vi "VMI_save_Files_backup.vi"(0 "appended path":path=path "C:/Users/Parkes/Documents/GitHub/Camera-Acquire_Labview/120416aa", 1 "ChangeFile":bool, 3 "Hist_full":dbl[][][](array[numeric]), 4 "Image Info":T1={"X size"=782.0, "Y size"=582.0, "Centroiding"=1.0}, 5 "Histogram_array":i32[][](array[numeric]), 6 "Current File Date":string, 7 "Remote Save?":bool, 9 "Collection Information":T3[](array[typedef]), 10 "Save":bool[](array[boolean]), 11 "error in (no error)":errorcluster, 12 "Remote_path":path=path "C:/Users/Parkes/Documents/GitHub/Camera-Acquire_Labview/120416aa", 13 "Peaks":T2[](array[typedef])) -> (8 "Remote_path\n 2":path[](array[path]), 15 "error out":errorcluster)   [LabVIEW 2020]
uses:
  Type defs/FileAcq_v1_Ctrl.ctl
  Type defs/VMI_peak_out.ctl
  Type defs/Image_info.ctl
  <vilib>/Utility/file.llb/Write Delimited Spreadsheet (string).vi
panel:
  out "size(s) 3":i32
  out "size(s) 2":i32[](array[numeric])
  out "size(s)":i32[](array[numeric])
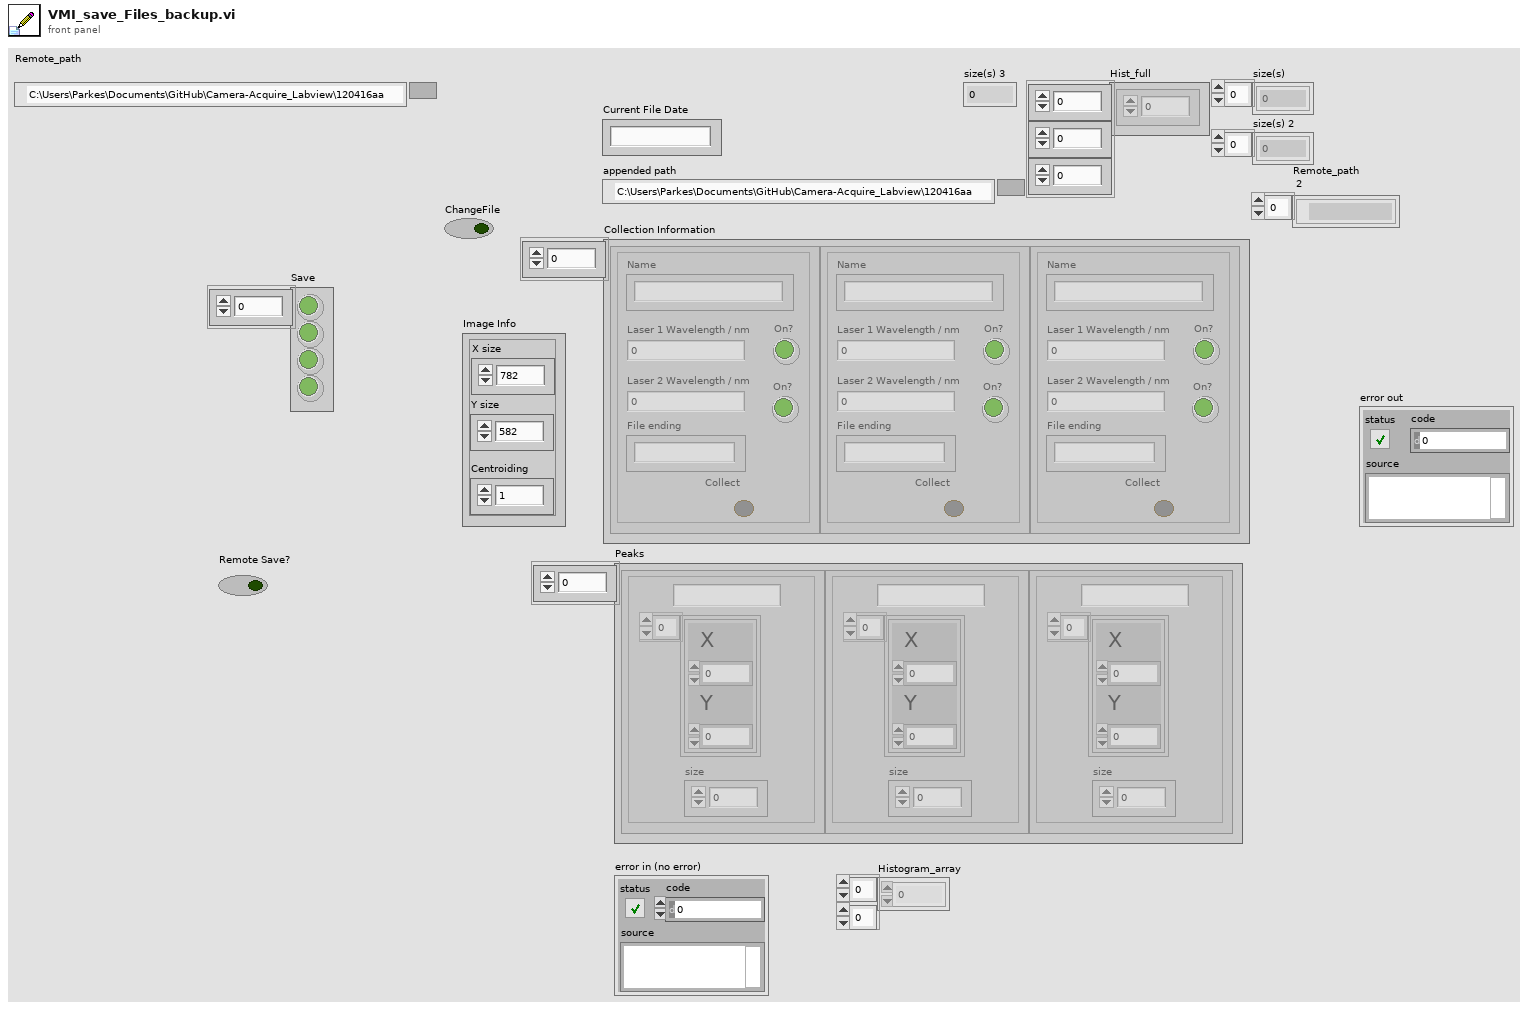
[diagram p1: front panel]
types:
  T1 = typedef "Image_info.ctl" = cluster{"X size":dbl, "Y size":dbl, "Centroiding":dbl}
  T2 = typedef "VMI_peak_out.ctl" = cluster{"Peaks":cluster{"X":sgl, "Y":sgl}[], "size":i32, "Title":string}
  T3 = typedef "FileAcq_v1_Ctrl.ctl" = cluster{"Type":string, "LaserWave1":dbl, "Shutter1":bool, "LaserWave2":dbl, "Shutter2":bool, "FileEnd":string, "Collect":bool}
  T4 = enum16{"open", "replace", "create", "open or create", "replace or create", "replace or create with confirmation"}
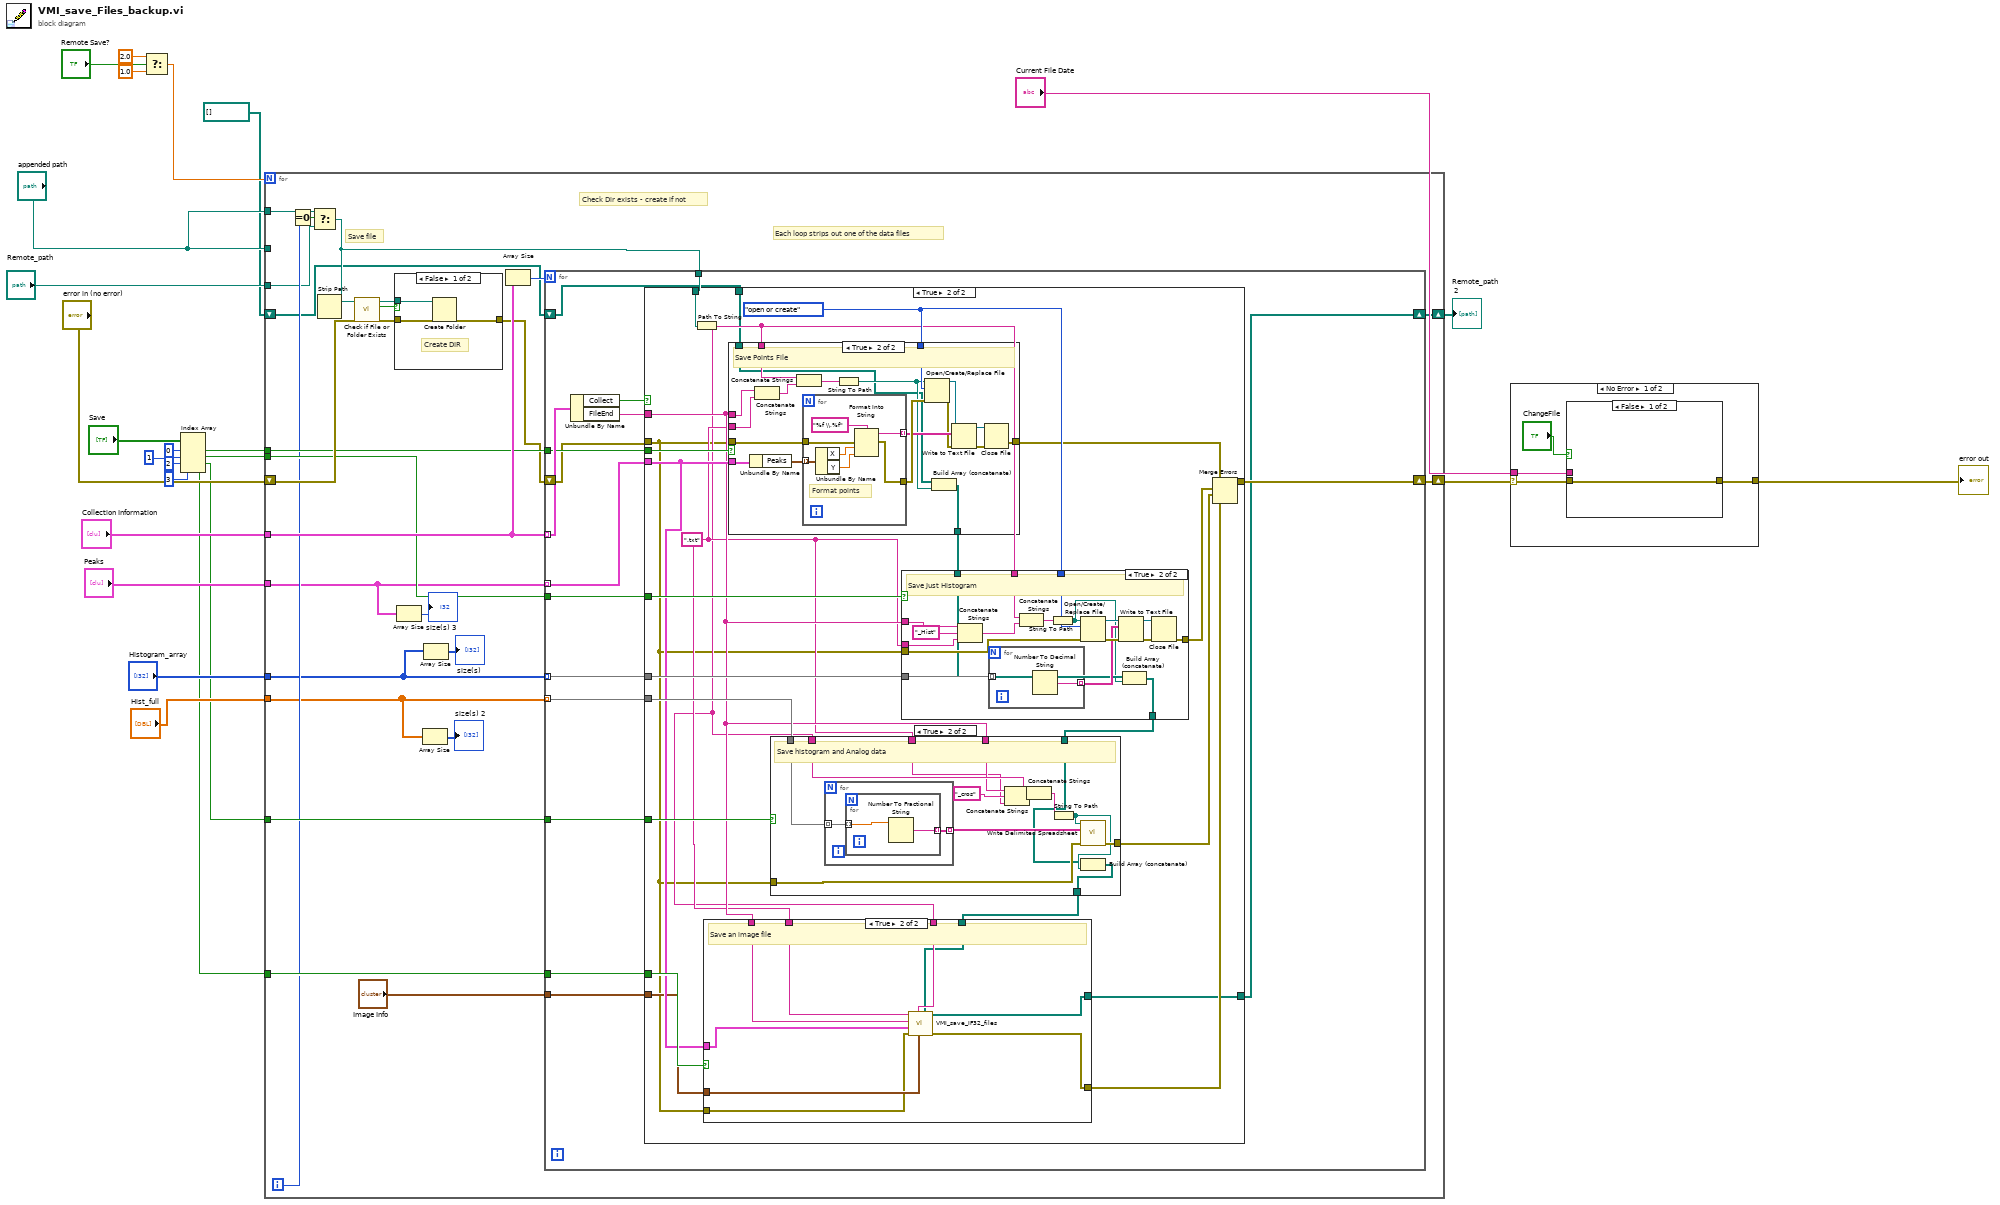
[diagram p0: block diagram]
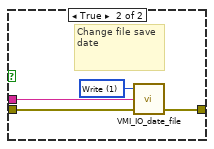
[diagram p8: hidden frame]
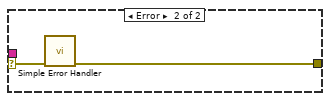
[diagram p9: hidden frame]
diagram:
  n1 = Select(t=2.0, s="Remote Save?", f=1.0) -> (s? t:f=w5:dbl)
  n2 = Index Array(array="Save", index #1=0 ("index"), index #2=1 ("index"), index #3=2 ("index"), index #4=3 ("index")) -> (element #1=w15:bool, element #2=w13:bool, element #3=w14:bool, element #4=w11:bool)
  n3 = for {
    N: w5 -> [_]
    tunnel: "appended path" -> [_]
    tunnel: "Histogram_array" -> [w32]
    tunnel: "Collection Information" -> [w45]
    tunnel: "Peaks" -> [w28]
    tunnel: "Hist_full" -> [w30]
    tunnel: w15 -> [w44]
    tunnel: w14 -> [w43]
    tunnel: w13 -> [w42]
    tunnel: w11 -> [w41]
    shift-right: [w38] -> w10
    shift-left: "error in (no error)" -> [w47]
    tunnel: "appended path" -> [w37]
    tunnel: "Remote_path" -> [w33]
    shift-right: [w26] -> w1
    shift-left: path[] [] ("Remote_path\n 2") -> [w25]
    i -> [w34]
    # "Each loop strips out one of the data files"
    # "Check Dir exists - create if not"
    # "Save file"
    n4 = Equal To 0?(x=w34) -> (x = 0?=w35:bool)
    n5 = Select(t=w37, s=w35, f=w33) -> (s? t:f=w36:path)
    n6 = Strip Path(path=w36) -> (stripped path=w51:path)  [unwired: 1 out]
    n7 = call <vilib>:"Check if File or Folder Exists.vi"("error in (no error)"=w47, "path"=w51) -> ("error out"=w48:errorcluster, "file or folder exists?"=w50:bool, "dup path"=w49:path)  [unwired: 7 in]
    n8 = case shown="False" w50 {
      tunnel: w49 -> [w54 _]
      tunnel: w48 -> [w53 w55]
      tunnel: [w52 w55] -> w39
      frame False {
        # "Create DIR"
        n9 = Create Folder(path (use dialog)=w54, error in=w53) -> (error out=w52:errorcluster)  [unwired: 1 in, 2 out]
      }
      frame True {
      }
    }
    n10 = Array Size(array=w28) -> (size(s)=→"size(s) 3":i32)
    n11 = Array Size(array=w30) -> (size(s)=→"size(s) 2":i32[])
    n12 = Array Size(array=w32) -> (size(s)=→"size(s)":i32[])
    n13 = Array Size(array=w45) -> (size(s)=w46:i32)
    n14 = for {
      N: w46 -> [_]
      tunnel: w45 -> [w69] mode=indexing
      tunnel: w36 -> [w71]
      tunnel: w32 -> [w70] mode=indexing
      tunnel: w28 -> [w65] mode=indexing
      tunnel: w30 -> [w66] mode=indexing
      tunnel: w44 -> [w64]
      tunnel: w43 -> [w63]
      tunnel: w42 -> [w62]
      tunnel: w41 -> [w61]
      tunnel: "Image Info" -> [w60]
      shift-right: [w58] -> w38
      shift-left: w39 -> [w59]
      shift-right: [w57] -> w26
      shift-left: w25 -> [w56]
      n15 = Unbundle By Name(w69) -> ("Collect"=w68:bool, "FileEnd"=w67:string)
      n16 = case shown="True" w68 {
        tunnel: w71 -> [_ w97]
        tunnel: [w73 w94] -> w58
        tunnel: w59 -> [w73 w80]
        tunnel: w70 -> [_ w96]
        tunnel: w67 -> [_ w83]
        tunnel: w66 -> [_ w93]
        tunnel: w65 -> [_ w85]
        tunnel: w64 -> [_ w88]
        tunnel: w63 -> [_ w89]
        tunnel: w62 -> [_ w87]
        tunnel: w61 -> [_ w86]
        tunnel: w60 -> [_ w84]
        tunnel: w56 -> [w72 w78]
        tunnel: [w72 w74] -> w57
        frame False {
        }
        frame True {
          w91 = T4."open or create" ("operation (0:open)")
          w82 = ".txt" ("string")
          n17 = Path To String(path=w97) -> (string=w81:string)
          n18 = case shown="True" w88 {
            tunnel: [w151 w155] -> w90
            tunnel: w80 -> [w151 w170]
            tunnel: w82 -> [_ w169]
            tunnel: w83 -> [_ w168]
            tunnel: w85 -> [_ w167]
            tunnel: w81 -> [_ w165]
            tunnel: w91 -> [_ w161]
            tunnel: w78 -> [w150 w153]
            tunnel: [w150 w152] -> w77
            frame False {
            }
            frame True {
              # "Save Points File"
              n19 = Unbundle By Name(w167) -> ("Peaks"=w166:cluster{"X":sgl, "Y":sgl}[])
              n20 = Concatenate Strings(w168, w169) -> (w164:string)
              n21 = Concatenate Strings(w165, w164) -> (w163:string)
              n22 = for {
                tunnel: w166 -> [w177] mode=indexing
                tunnel: [w173] -> w159 mode=indexing
                tunnel: [w172] -> w162
                tunnel: w170 -> [w171]
                # "Format points"
                n23 = Unbundle By Name(w177) -> ("X"=w176:sgl, "Y"=w175:sgl)
                n24 = Format Into String(format string="%f \\,%f", error in=w171, w176, w175) -> (resulting string=w173:string, error out=w172:errorcluster)  [unwired: 1 in]
              }
              n25 = String To Path(string=w163) -> (path=w154:path)
              n26 = Open/Create/Replace File(file path (use dialog)=w154, error in=w162, operation (0:open)=w161) -> (refnum out=w160:refnum<file>, error out=w158:errorcluster)  [unwired: 3 in, 1 out]
              n27 = Build Array (concatenate)(w153, w154) -> (w152:path[])
              n28 = Write to Text File(file (use dialog)=w160, text=w159, error in=w158) -> (refnum out=w157:refnum<file>, error out=w156:errorcluster)  [unwired: 1 in, 1 out]
              n29 = Close File(refnum=w157, error in=w156) -> (error out=w155:errorcluster)  [unwired: 1 out]
            }
          }
          n30 = case shown="True" w87 {
            tunnel: w82 -> [_ w127]
            tunnel: w96 -> [_ w122]
            tunnel: [w110 w114] -> w95
            tunnel: w81 -> [_ w120]
            tunnel: w91 -> [_ w119]
            tunnel: w83 -> [_ w118]
            tunnel: w80 -> [w110 w117]
            tunnel: w77 -> [w109 w113]
            tunnel: [w109 w111] -> w76
            frame False {
            }
            frame True {
              # "Save Just Histogram"
              n31 = Concatenate Strings(w118, "_Hist" ("string"), w127) -> (w126:string)
              n32 = for {
                tunnel: w122 -> [w130] mode=indexing
                tunnel: [w129] -> w121 mode=indexing
                n33 = Number To Decimal String(number=w130) -> (decimal integer string=w129:string)  [unwired: 1 in]
              }
              n34 = Concatenate Strings(w120, w126) -> (w125:string)
              n35 = String To Path(string=w125) -> (path=w112:path)
              n36 = Open/Create/Replace File(file path (use dialog)=w112, error in=w117, operation (0:open)=w119) -> (refnum out=w124:refnum<file>, error out=w123:errorcluster)  [unwired: 3 in, 1 out]
              n37 = Write to Text File(file (use dialog)=w124, text=w121, error in=w123) -> (refnum out=w116:refnum<file>, error out=w115:errorcluster)  [unwired: 1 in, 1 out]
              n38 = Build Array (concatenate)(w113, w112) -> (w111:path[])
              n39 = Close File(refnum=w116, error in=w115) -> (error out=w114:errorcluster)  [unwired: 1 out]
            }
          }
          n40 = case shown="True" w89 {
            tunnel: w93 -> [_ w145]
            tunnel: [w132 w140] -> w92
            tunnel: w81 -> [_ w139]
            tunnel: w83 -> [_ w138]
            tunnel: w80 -> [w132 w136]
            tunnel: w82 -> [_ w137]
            tunnel: w76 -> [w131 w134]
            tunnel: [w131 w133] -> w75
            frame False {
            }
            frame True {
              # "Save histogram and Analog data"
              n41 = for {
                tunnel: w145 -> [w147] mode=indexing
                tunnel: [w146] -> w144 mode=indexing
                n42 = for {
                  tunnel: w147 -> [w149] mode=indexing
                  tunnel: [w148] -> w146 mode=indexing
                  n43 = Number To Fractional String(number=w149) -> (F-format string=w148:string)  [unwired: 3 in]
                }
              }
              n44 = Concatenate Strings(w138, "_cros" ("string"), w137) -> (w142:string)
              n45 = Concatenate Strings(w139, w142) -> (w141:string)
              n46 = String To Path(string=w141) -> (path=w135:path)
              n47 = call-poly <vilib>:"Write Delimited Spreadsheet.vi"("file path (dialog if empty)"=w135, "2D data"=w144, "error in (no error)"=w136) -> ("error out"=w140:errorcluster)  [unwired: 11 in, 1 out]
              n48 = Build Array (concatenate)(w134, w135) -> (w133:path[])
            }
          }
          n49 = case shown="True" w86 {
            tunnel: w85 -> [_ w108]
            tunnel: w84 -> [_ w107]
            tunnel: w83 -> [_ w106]
            tunnel: w82 -> [_ w105]
            tunnel: w81 -> [_ w104]
            tunnel: w80 -> [w99 w103]
            tunnel: [w99 w102] -> w79
            tunnel: w75 -> [w98 w101]
            tunnel: [w98 w100] -> w74
            frame False {
            }
            frame True {
              # "Save an image file"
              n50 = call "VMI_save_IF32_files.vi"("Remote_path\n in"=w101, "Image Info"=w107, "file_path"=w104, "error in (no error)"=w103, "Peak Controls"=w108, "FileEnd"=w106, "file ending"=w105) -> ("error out"=w102:errorcluster, "Array"=w100:path[])  [unwired: 3 in]
            }
          }
          n51 = Merge Errors(w90, w95, w92, w79) -> (w94:errorcluster)
        }
      }
    }
  }
  "error out" <- w10
  "Remote_path\n 2" <- w1
  n52 = case shown="No Error" w10 {
    selector: w10 -> [w180 w188]
    tunnel: "Current File Date" -> [w181 _]
    tunnel: [w179 w187] -> _
    frame No Error {
      n53 = case shown="False" "ChangeFile" {
        tunnel: w181 -> [_ w186]
        tunnel: w180 -> [w182 w185]
        tunnel: [w182 w183] -> w179
        frame False {
        }
        frame True {
          w184 = u16 1 items=["Read", "Write"] ("File Task")
          # "Change file save\ndate"
          n54 = call "VMI_IO_date_file.vi"("Error In"=w185, "File date in"=w186, "File Task"=w184) -> ("Error Out"=w183:errorcluster)  [unwired: 1 in, 1 out]
        }
      }
    }
    frame Error {
      n55 = call <vilib>:"Simple Error Handler.vi"("error in (no error)"=w188) -> ("error out"=w187:errorcluster)  [unwired: 4 in, 4 out]
    }
  }
